vi "Write Verify Server.vi"(8 "error in (no error)":errorcluster, 10 "Verify Server":bool=TRUE, 11 "REST Client in":refnum<class "REST Client.lvclass">) -> (0 "error out":errorcluster, 3 "REST Client out":refnum<class "REST Client.lvclass">)   [LabVIEW 2013, in "REST Client.lvlib" / "REST Client.lvclass"]
doc: "Write Verify Server"
uses:
  REST Client.lvclass
  REST Client.lvclass/REST Client.ctl
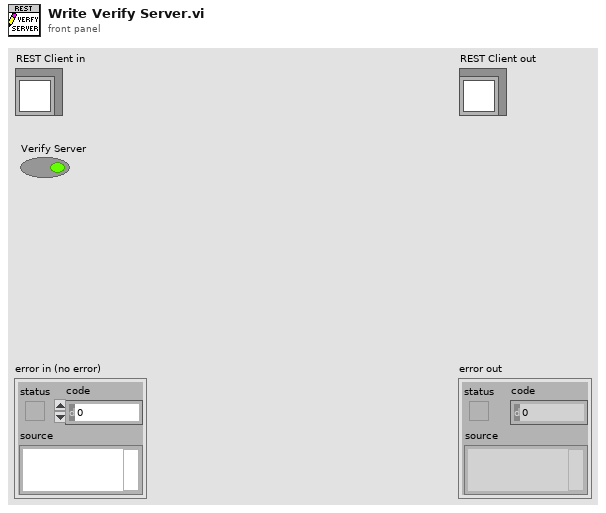
[diagram p1: front panel]
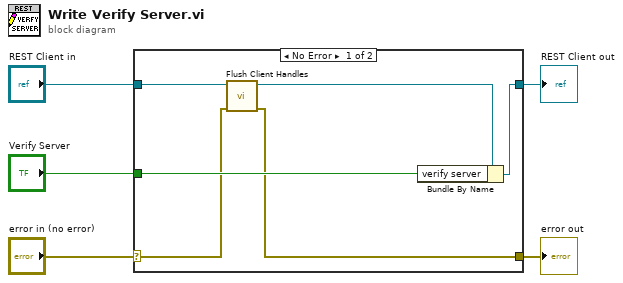
[diagram p0: block diagram]
diagram:
  n1 = case shown="No Error" "error in (no error)" {
    selector: "error in (no error)" -> [w8 w12]
    tunnel: [w7 w12] -> w4
    tunnel: [w11 w13] -> w2
    tunnel: "REST Client in" -> [w9 w13]
    tunnel: "Verify Server" -> [w10 _]
    frame No Error {
      n2 = call-dynamic "Flush Client Handles.vi"("error in (no error)"=w8, "REST Client in"=w9) -> ("error out"=w7:errorcluster, "REST Client out"=w6:refnum<class "REST Client.lvclass">)  [unwired: 8 in]
      n3 = Bundle By Name(cluster=w6, "verify server"=w10) -> (w11:refnum<class "REST Client.lvclass">)
    }
    frame Error {
    }
  }
  "error out" <- w4
  "REST Client out" <- w2
